vi "Logarithm Color Ramp.vi"(4 "Bottom Numeric":sgl, 5 "Logarithm?":bool, 6 "Top Numeric":sgl, 8 "error in (no error)":errorcluster, 9 "Numeric Ref Array":refnum<vi>[](array[refnum]), 10 "Color Ref Array":refnum<vi>[](array[refnum]), 11 "Slider Ref Array":refnum<vi>[](array[refnum])) -> (0 "error out":errorcluster)   [LabVIEW 2020, in "3D Plot.lvclass"]
uses:
  <vilib>/Math Plots/3D Math Plots/3D Plot/3D Plot/3D Plot.lvclass
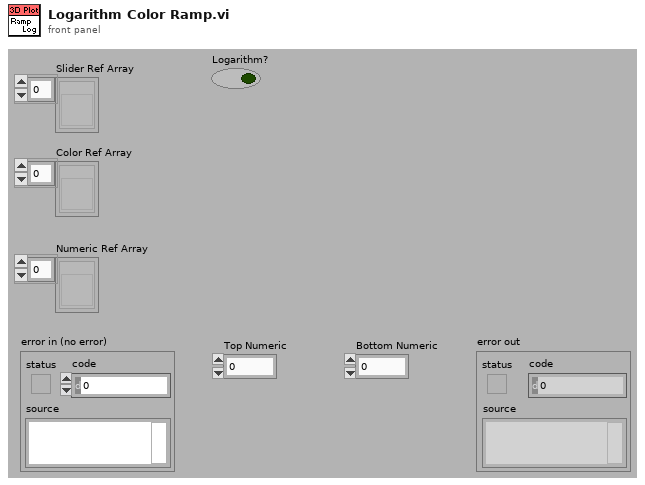
[diagram p1: front panel]
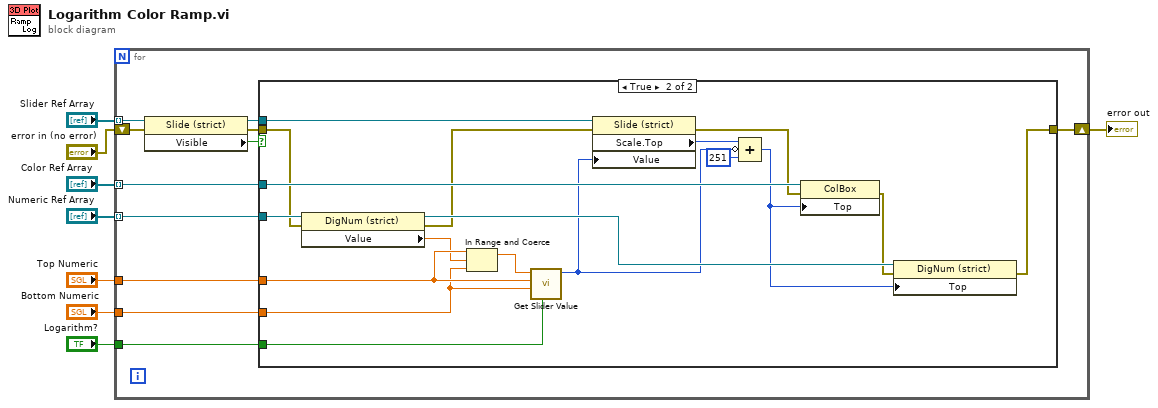
[diagram p0: block diagram]
diagram:
  n1 = for {
    tunnel: "Slider Ref Array" -> [w19] mode=indexing
    tunnel: "Numeric Ref Array" -> [w17] mode=indexing
    tunnel: "Color Ref Array" -> [w16] mode=indexing
    tunnel: "Top Numeric" -> [w15]
    tunnel: "Bottom Numeric" -> [w14]
    tunnel: "Logarithm?" -> [w12]
    shift-right: [w10] -> w1
    shift-left: "error in (no error)" -> [w9]
    n2 = property class="Slide (strict)"(reference=w19, error in=w9) -> (reference out=w13:refnum<vi>, error out=w11:errorcluster, "Visible"=w18:bool)
    n3 = case shown="True" w18 {
      tunnel: w17 -> [_ w38]
      tunnel: w16 -> [_ w30]
      tunnel: w15 -> [_ w36]
      tunnel: w14 -> [_ w35]
      tunnel: w13 -> [_ w31]
      tunnel: w12 -> [_ w28]
      tunnel: w11 -> [w20 w27]
      tunnel: [w20 w22] -> w10
      frame False {
      }
      frame True {
        n4 = property class="DigNum (strict)"(reference=w38, error in=w27) -> (reference out=w29:refnum<vi>, error out=w26:errorcluster, "Value"=w34:sgl)
        n5 = In Range and Coerce(upper limit=w36, x=w34, lower limit=w35) -> (coerced(x)=w37:sgl)  [unwired: 1 out]
        n6 = call <vilib>:"Get Slider Value.vi"("Logarithm?"=w28, "Bottom Numeric"=w35, "Top Numeric"=w36, "Current Numeric"=w37) -> ("Current Slider"=w21:i32)  [unwired: 7 out]
        n7 = property class="Slide (strict)"(reference=w31, error in=w26, "Value"=w21) -> (error out=w24:errorcluster, "Scale.Top"=w33:i32)  [unwired: 1 out]
        n8 = Compound Arithmetic op=ADD(w33, invert w21, 251 ("value")) -> (w25:i32)
        n9 = property class="ColBox"(reference=w30, error in=w24, "Top"=w25) -> (error out=w23:errorcluster)  [unwired: 1 out]
        n10 = property class="DigNum (strict)"(reference=w29, error in=w23, "Top"=w25) -> (error out=w22:errorcluster)  [unwired: 1 out]
      }
    }
  }
  "error out" <- w1
